vi "DIDs.vi"(8 "error in (no error)":errorcluster, 11 "Node Ptr":T1 format="%.0x") -> (0 "error out":errorcluster)   [LabVIEW 2013, in "Diagnostics Addon System Explorer.lvlib"]
uses:
  Diagnostics Addon System Explorer.lvlib
  <vilib>/NI Veristand/Custom Device API/Custom Device Item Ref.ctl
  Shared/FG Action.ctl
  Shared/GUID Lookup.vi
  <vilib>/NI Veristand/Custom Device API/NI VeriStand - Get Item Property.vi
  <vilib>/NI Veristand/Custom Device API/Get Item Property (Variant).vi
  <vilib>/NI Veristand/Custom Device API/Custom Device API.lvlib
  Shared/Diagnostics Addon Shared.lvlib
panel:
  in  "SHDocVw.IWebBrowser":refnum<k7>(container)
  out "Channels":i32(listbox)
  in  "Description":string
  out "Name":string
  in  "Header":cluster{"Section Name":string}={"Section Name"="Custom Device Item Settings"}
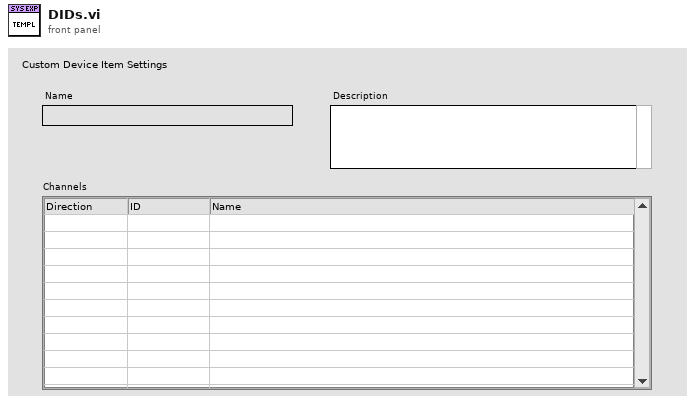
[diagram p1: front panel]
types:
  T1 = typedef "Custom Device API.lvlib/Custom Device Item Ref.ctl" = u64
  T2 = typedef "Diagnostics Addon Shared.lvlib/FG Action.ctl" = enum16{"Get", "Set"}
  T3 = typedef "Custom Device API.lvlib/Custom Device Item Info.ctl" = cluster{"Name":string, "Is Channel":bool, "GUID":string, "Is Waveform":bool}
  T4 = typedef "Custom Device API.lvlib/Custom Device Commands.ctl" = enum16{"Default", "Item renamed", "Shutdown", "Dynamic button pressed"}
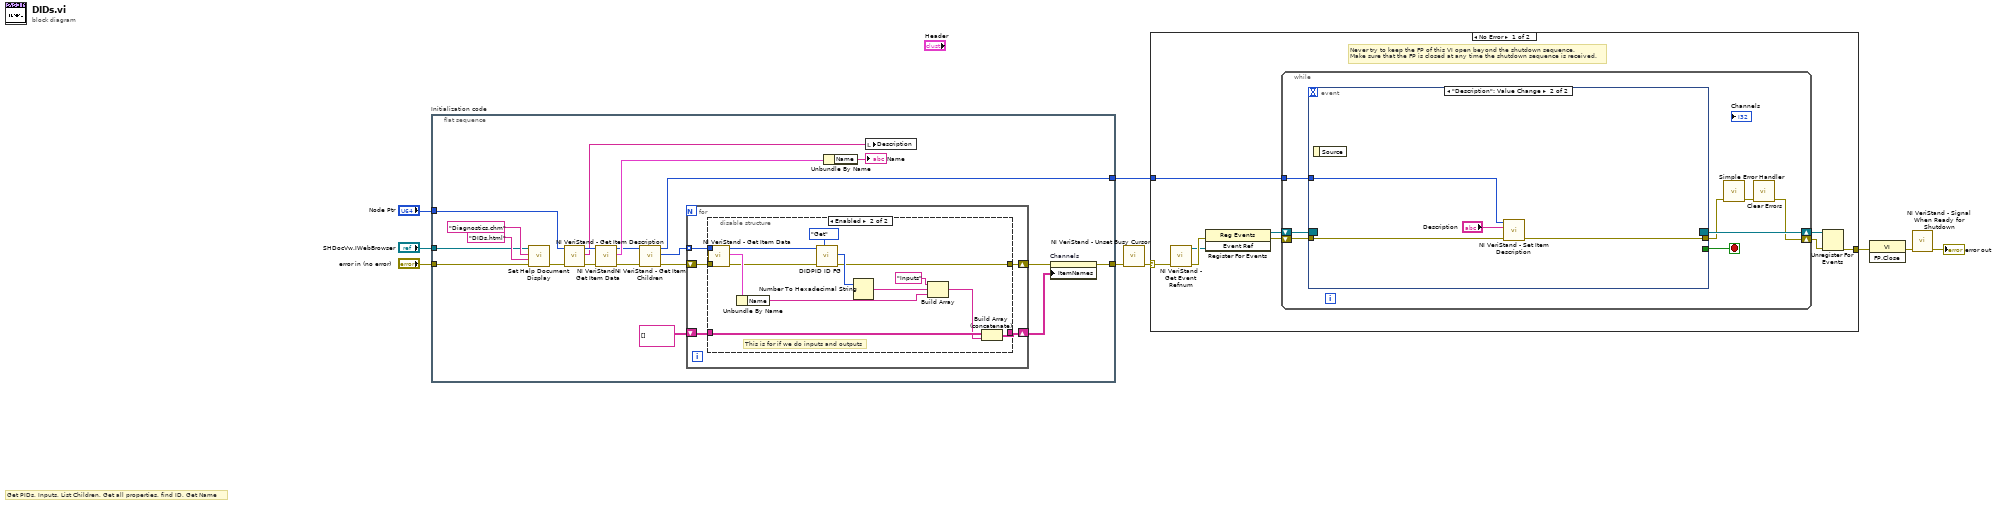
[diagram p0: block diagram]
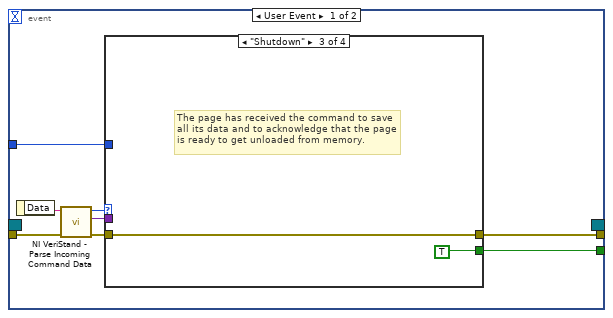
[diagram p2: hidden frame]
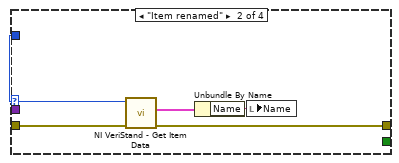
[diagram p4: hidden frame]
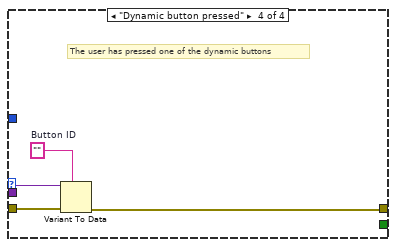
[diagram p5: hidden frame]
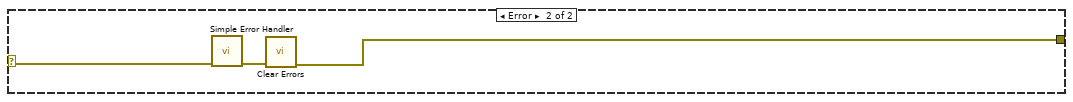
[diagram p6: hidden frame]
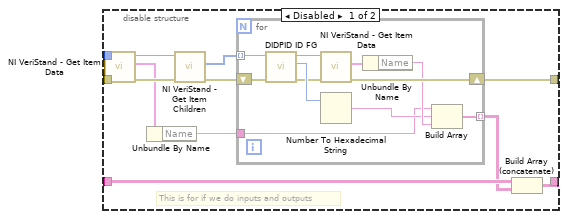
[diagram p7: hidden frame]
diagram:
  # "Get PIDs, Inputs, List Children, Get all properties, find ID, Get Name"
  n1 = flat-sequence "Initialization code" {
    tunnel: "error in (no error)" -> [w22]
    tunnel: "Node Ptr" -> [w28]
    tunnel: [w18] -> w5
    tunnel: [w14] -> w2
    tunnel: "SHDocVw.IWebBrowser" -> [w20]
    frame #0 {
      n2 = call "Set Help Document Display.vi"("error in (no error)"=w22, "HTML File"="DIDs.html", "Main CHM File"="Diagnostics.chm", "SHDocVw.IWebBrowser2"=w20) -> ("error out"=w21:errorcluster)  [unwired: 7 in]
      n3 = call <vilib>:"NI VeriStand - Get Item Description.vi"("error in (no error)"=w21, "Item Ref in"=w28) -> ("error out"=w26:errorcluster, "Description"=w27:string, "Item Ref out"=w29:T1)  [unwired: 7 out]
      n4 = call <vilib>:"NI VeriStand - Get Item Data.vi"("error in (no error)"=w26, "Item Ref in"=w29) -> ("error out"=w17:errorcluster, "Item Info"=w25:T3, "Item Ref out"=w16:T1)  [unwired: 7 out]
      n5 = call <vilib>:"NI VeriStand - Get Item Children.vi"("error in (no error)"=w17, "Item Ref in"=w16) -> ("error out"=w15:errorcluster, "Child Refs"=w13:T1[], "Item Ref out"=w14:T1)  [unwired: 6 in, 1 out]
      n6 = for {
        tunnel: w13 -> [w32] mode=indexing
        shift-right: [w34] -> w19
        shift-left: w15 -> [w33]
        shift-right: [w30] -> w11
        shift-left: string[][] [] -> [w31]
        n7 = disable-structure shown="Enabled" {
          disable-tunnel: [w46 w60] -> w34
          disable-tunnel: w33 -> [w43 w71]
          disable-tunnel: w32 -> [w38 w69]
          disable-tunnel: w31 -> [w37 w68]
          disable-tunnel: [w35 w66] -> w30
          frame Disabled {
            # "This is for if we do inputs and outputs"
            n8 = call <vilib>:"NI VeriStand - Get Item Data.vi"("error in (no error)"=w43, "Item Ref in"=w38) -> ("error out"=w42:errorcluster, "Item Info"=w40:T3, "Item Ref out"=w41:T1)  [unwired: 7 out]
            n9 = Unbundle By Name(w40) -> ("Name"=w39:string)
            n10 = call <vilib>:"NI VeriStand - Get Item Children.vi"("error in (no error)"=w42, "Item Ref in"=w41) -> ("error out"=w44:errorcluster, "Child Refs"=w45:T1[])  [unwired: 6 in, 2 out]
            n11 = for {
              tunnel: w45 -> [w57] mode=indexing
              shift-right: [w53] -> w46
              shift-left: w44 -> [w56]
              tunnel: [w48] -> w36 mode=indexing
              tunnel: w39 -> [w47]
              n12 = call "DIDPID ID FG.vi"("error in (no error)"=w56, "Device Item Ref in"=w57) -> ("error out"=w54:errorcluster, "ID"=w55:u16, "Device Item Ref out"=w52:T1)  [unwired: 7 in]
              n13 = call <vilib>:"NI VeriStand - Get Item Data.vi"("error in (no error)"=w54, "Item Ref in"=w52) -> ("error out"=w53:errorcluster, "Item Info"=w51:T3)  [unwired: 8 out]
              n14 = Number To Hexadecimal String(2:w55) -> (0:w49:string)  [unwired: 1 in]
              n15 = Unbundle By Name(w51) -> ("Name"=w50:string)
              n16 = Build Array(w47, w49, w50) -> (w48:string[])
            }
            n17 = Build Array (concatenate)(w37, w36) -> (w35:string[][])
          }
          frame Enabled {
            # "This is for if we do inputs and outputs"
            n18 = call <vilib>:"NI VeriStand - Get Item Data.vi"("error in (no error)"=w71, "Item Ref in"=w69) -> ("error out"=w63:errorcluster, "Item Info"=w70:T3, "Item Ref out"=w62:T1)  [unwired: 7 out]
            n19 = Unbundle By Name(w70) -> ("Name"=w61:string)
            n20 = call "DIDPID ID FG.vi"("Action"=FG_Action."Get", "error in (no error)"=w63, "Device Item Ref in"=w62) -> ("error out"=w60:errorcluster, "ID"=w65:u16)  [unwired: 6 in, 1 out]
            n21 = Number To Hexadecimal String(2:w65) -> (0:w64:string)  [unwired: 1 in]
            n22 = Build Array("Inputs" ("element"), w64, w61) -> (w67:string[])
            n23 = Build Array (concatenate)(w68, w67) -> (w66:string[][])
          }
        }
      }
      n24 = Unbundle By Name(w25) -> ("Name"=→"Name":string)
      n25 = local write "Description"(w27) -> ()
      n26 = property on="Channels" class="MCListbox (strict)"(error in=w19, "ItemNames"=w11) -> (error out=w18:errorcluster)  [unwired: 1 in, 1 out]
    }
  }
  n27 = call <vilib>:"NI VeriStand - Unset Busy Cursor.vi"("error in (no error)"=w5) -> ("error out"=w4:errorcluster)  [unwired: 10 out]
  n28 = case shown="No Error" w4 {
    selector: w4 -> [w72 w115]
    tunnel: [w77 w113] -> w9
    tunnel: w2 -> [w73 _]
    frame No Error {
      # "Never try to keep the FP of this VI open beyond the shutdown sequence.\nMake sure that the FP is closed at any time the shutdown sequence is received."
      n29 = call <vilib>:"NI VeriStand - Get Event Refnum.vi"("error in (no error)"=w72) -> ("error out"=w80:errorcluster, "Event Ref"=w76:refnum<user-event>)  [unwired: 9 out]
      n30 = register-events(error in=w80, w76) -> (reference out=w74:refnum<event-registration>, error out=w75:errorcluster)  [unwired: 1 in]
      n31 = while {
        tunnel: w73 -> [w84]
        shift-right: [w81] -> w78
        shift-left: w75 -> [w87]
        shift-right: [w88] -> w79
        shift-left: w74 -> [w86]
        stop <- w85 stop-if-true
        n32 = event shown="[1] \"Description\": Value Change" {
          selector: w86 -> [_ _]
          dyn-events: [_ _] -> w88
          timeout: _ -> [_ _]
          tunnel: w87 -> [w96 w111]
          tunnel: [w92 _] -> w85
          tunnel: [w91 w110] -> w83
          tunnel: w84 -> [w90 w112]
          event User Event {
            n33 = event-data() -> ("Data"=w95:string)  [unwired: 1 out]
            n34 = call <vilib>:"NI VeriStand - Parse Incoming Command Data.vi"("error in (no error)"=w96, "Incoming data"=w95) -> ("error out"=w94:errorcluster, "Outgoing data"=w89:variant, "Action"=w93:T4)  [unwired: 7 out]
            n35 = case shown="\"Shutdown\"" w93 {
              tunnel: w94 -> [w97 w102 w103 w108]
              tunnel: [_ _ TRUE _] -> w92
              tunnel: [w97 w99 w103 w105] -> w91
              tunnel: w90 -> [_ w101 _ _]
              tunnel: w89 -> [_ _ _ w107]
              frame "Default", Default {
              }
              frame "Item renamed" {
                n36 = call <vilib>:"NI VeriStand - Get Item Data.vi"("error in (no error)"=w102, "Item Ref in"=w101) -> ("error out"=w99:errorcluster, "Item Info"=w100:T3)  [unwired: 8 out]
                n37 = Unbundle By Name(w100) -> ("Name"=w98:string)
                n38 = local write "Name"(w98) -> ()
              }
              frame "Shutdown" {
                # "The page has received the command to save all its data and to acknowledge that the page is ready to get unloaded from memory."
              }
              frame "Dynamic button pressed" {
                w106 = ""  # Button ID
                # "The user has pressed one of the dynamic buttons"
                n39 = Variant To Data(error in=w108, type=w106, Variant=w107) -> (error out=w105:errorcluster)  [unwired: 1 out]
              }
            }
          }
          event "Description": Value Change {
            n40 = event-data() -> ()  [unwired: 2 out]
            n41 = call <vilib>:"NI VeriStand - Set Item Description.vi"("error in (no error)"=w111, "Description"="Description", "Item Ref in"=w112) -> ("error out"=w110:errorcluster)  [unwired: 8 out]
          }
        }
        n42 = call <vilib>:"Simple Error Handler.vi"("error in (no error)"=w83) -> ("error out"=w82:errorcluster)  [unwired: 1 in, 7 out]
        n43 = call <vilib>:"Clear Errors.vi"("error in (no error)"=w82) -> ("error out"=w81:errorcluster)  [unwired: 6 out]
      }
      n44 = Unregister For Events(event registration refnum=w79, error in=w78) -> (error out=w77:errorcluster)
    }
    frame Error {
      n45 = call <vilib>:"Simple Error Handler.vi"("error in (no error)"=w115) -> ("error out"=w114:errorcluster)  [unwired: 1 in, 7 out]
      n46 = call <vilib>:"Clear Errors.vi"("error in (no error)"=w114) -> ("error out"=w113:errorcluster)  [unwired: 6 out]
    }
  }
  n47 = invoke class="VI" method="FP.Close"(error in=w9) -> (error out=w8:errorcluster)  [unwired: 2 in, 2 out]
  n48 = call <vilib>:"NI VeriStand - Signal When Ready for Shutdown.vi"("error in (no error)"=w8) -> ("error out"=→"error out":errorcluster)  [unwired: 10 out]
